vi "TestVisionSavedImage.vi"() -> ()   [LabVIEW 2019]
uses:
  <vilib>/vision/NI_Vision_Development_Module.lvlib
panel:
  out "Real World Coordinates":cluster{"X":sgl, "Y":sgl} {"Y" format="%.2f"; "X" format="%.2f"}
  out "Length":dbl
  out "Valid Coordinates":bool
  out "End Y":i32
  out "End X":i32
  out "Start Y":i32
  out "Start X":i32
  out "Line":T1 {"Start X" scale=0.0..1024.0; "End X" scale=0.0..1024.0}
  in  "File Path":path
  out "Image":T2(plugin-control)
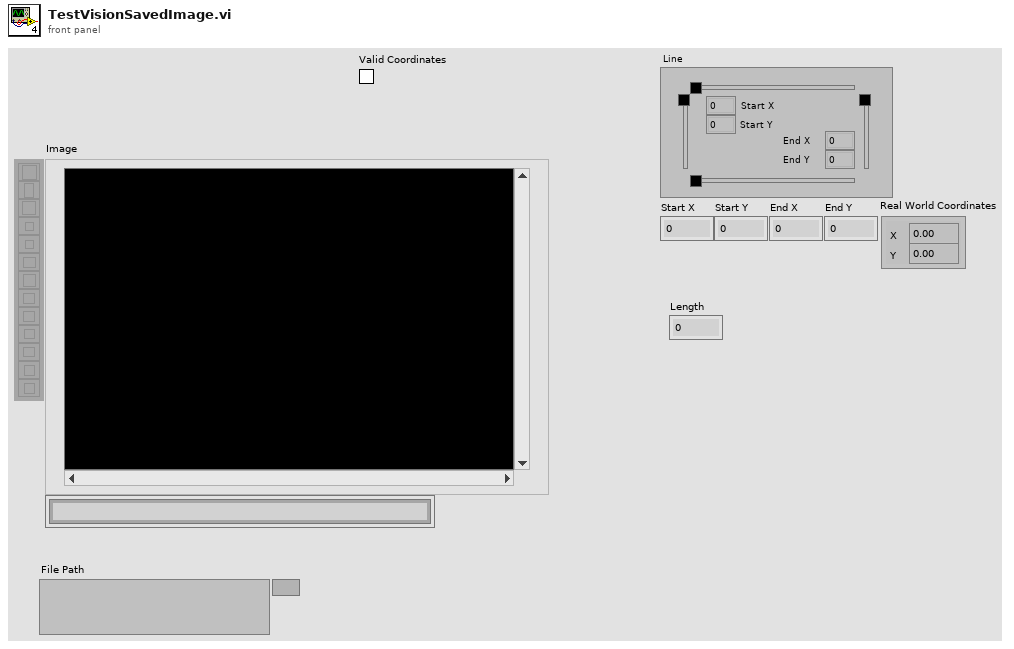
[diagram p1: front panel]
types:
  T1 = typedef "IMAQ Line" = cluster{"Start X":i32, "Start Y":i32, "End X":i32, "End Y":i32}
  T2 = typedef "IMAQ Image.ctl" = refnum<image>
  T3 = typedef "Simple Grid Descriptor" = cluster{"X Step":sgl, "Y Step":sgl, "Unit":T4}
  T4 = typedef "Image Unit" = enum32{"Undefined", "Angström", "Micrometer", "Millimeter", "Centimeter", "Meter", "Kilometer", "Microinch", "Inch", "Feet", "Nautical miles", "Standard miles", "Steps"}
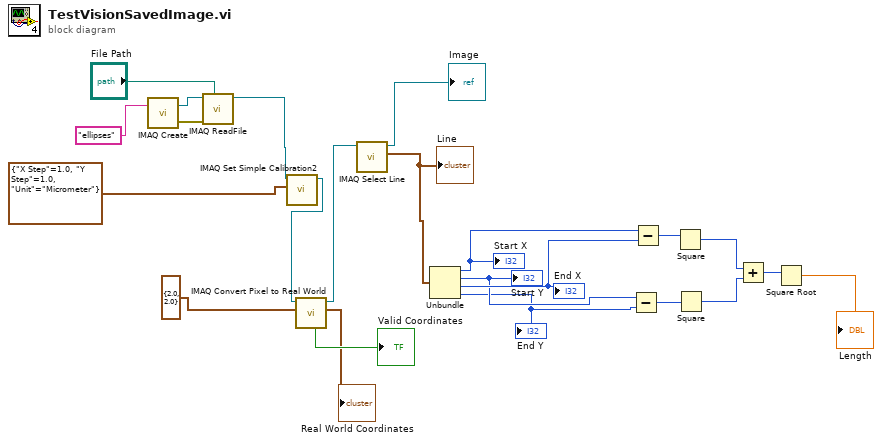
[diagram p0: block diagram]
diagram:
  n1 = call "IMAQ Create"("Image Name"="ellipses") -> ("New Image"=w21:T2, "error out"=w20:errorcluster)  [unwired: 4 in]
  n2 = call "IMAQ ReadFile"("File Path"="File Path", "error in (no error)"=w20, "Image"=w21) -> ("Image Out"=w2:T2)  [unwired: 4 in, 4 out]
  n3 = call "IMAQ Set Simple Calibration2"("Pixel Distances"=T3 {"X Step"=1.0, "Y Step"=1.0, "Unit"=enum."Micrometer"}, "Image"=w2) -> ("Calibration Template Image"=w1:T2)  [unwired: 8 in, 1 out]
  n4 = call "IMAQ Convert Pixel to Real World"("Pixel Coordinates"=cluster{"X":sgl, "Y":sgl} {"X"=2.0, "Y"=2.0}, "Calibrated Image"=w1) -> ("Real World Coordinates"=→"Real World Coordinates":cluster{"X":sgl, "Y":sgl}, "Calibrated Image (duplicate)"=w15:T2, "Valid Coordinates"=→"Valid Coordinates":bool)  [unwired: 4 in, 3 out]
  n5 = call "IMAQ Select Line"("Image In"=w15) -> ("Line"=w18:T1, "Image Out (duplicate)"=→"Image":T2)  [unwired: 7 in, 2 out]
  "Line" <- w18
  n6 = Unbundle(w18) -> ("Start X"=w13:i32, "Start Y"=w10:i32, "End X"=w12:i32, "End Y"=w9:i32)
  "Start X" <- w13
  "Start Y" <- w10
  "End X" <- w12
  "End Y" <- w9
  n7 = Subtract(x=w10, y=w9) -> (x-y=w8:i32)
  n8 = Subtract(x=w13, y=w12) -> (x-y=w11:i32)
  n9 = Square(x=w11) -> (x^2=w7:i32)
  n10 = Square(x=w8) -> (x^2=w6:i32)
  n11 = Add(x=w7, y=w6) -> (x+y=w5:i32)
  n12 = Square Root(x=w5) -> (sqrt(x)=→"Length":dbl)
